vi "Write_para_port2_singalChange.vi"(8 "error in (no error)":errorcluster caption="错误输入（无错误）", 9 "索引":i32, 10 "布尔":bool=TRUE, 11 "address":i16=888 caption="地址" format="%.0x") -> (0 "error out":errorcluster caption="错误输出")   [LabVIEW 2011]
uses:
  <vilib>/Platform/portaccess.llb/In Port8.vi
  <vilib>/Platform/portaccess.llb/Out Port32.vi
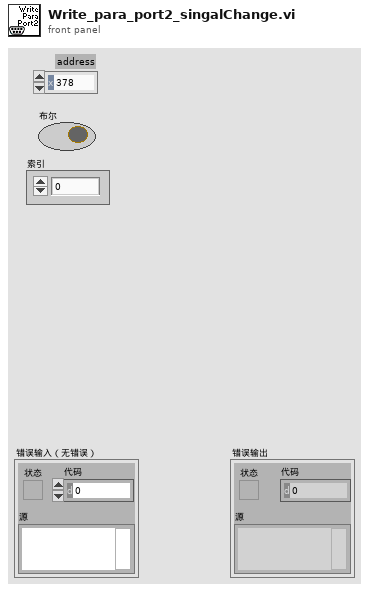
[diagram p1: front panel]
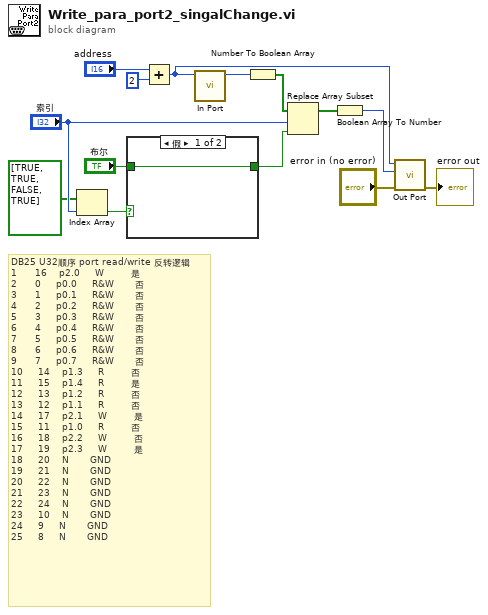
[diagram p0: block diagram]
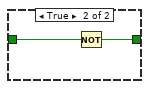
[diagram p2: hidden frame]
diagram:
  # "DB25\tU32顺序\tport\tread/write\t反转逻辑\n1\t     16\t   p2.0    \tW\t        是\n2\t     0    \tp0.0\t   \tR&W\t      否\n3\t     1\t\t   p0.1\t   \tR&W      \t否\n4\t\t    2\t   \tp0.2   \t\tR&W      \t否\n5\t\t    3\t\t   p0.3   \t\tR&W\t      否\n6\t\t    4\t   \tp0.4   \t\tR&W      \t否\n7\t\t    5\t   \tp0.5   \t\tR&W      \t否\n8\t\t    6\t   \tp0.6\t   \tR&W      \t否\n9\t    \t7\t   \tp0.7\t   \tR&W\t      否\n10\t    14   \tp1.3   \t\tR        \t否\n11\t   \t15   \tp1.4   \t\tR        \t是\n12\t   \t13   \tp1.2\t   \tR        \t否\n13    \t12   \tp1.1\t   \tR        \t否\n14     17   \tp2.1\t   \tW        \t是\n15    \t11   \tp1.0   \t\tR\t        否\n16    \t18   \tp2.2   \t\tW        \t否\n17    \t19\t   p2.3   \t\tW\t        是\n18    \t20   \tN   \t  \tGND\t\n19    \t21   \tN   \t  \tGND\t\n20\t    22\t   N\t  \t  \tGND\t\n21\t    23\t   N  \t  \t\tGND\t\n22\t    24\t   N  \t  \t\tGND\t\n23    \t10   \tN  \t  \t\tGND\t\n24    \t9\t    N  \t  \t\tGND\t\n25\t    8    \tN  \t  \t\tGND"
  n1 = Index Array(array=bool[] [TRUE, TRUE, FALSE, TRUE], index="索引") -> (element=w2:bool)
  n2 = case shown="假" w2 {
    tunnel: "布尔" -> [w15 w17]
    tunnel: [w15 w16] -> w1
    frame False {
    }
    frame True {
      n3 = Not(x=w17) -> (.not. x?=w16:bool)
    }
  }
  n4 = Add(x="address", y=i16 2) -> (x+y=w6:i16)
  n5 = call-poly <vilib>:"In Port.vi"("address"=w6) -> ("data read"=w12:i8)  [unwired: 7 in, 1 out]
  n6 = Number To Boolean Array(number=w12) -> (Boolean array=w11:bool[])
  n7 = Replace Array Subset(array=w11, new element=w1, index="索引") -> (w10:bool[])
  n8 = Boolean Array To Number(Boolean array=w10) -> (number=w9:u32)
  n9 = call-poly <vilib>:"Out Port.vi"("error in (no error)"="error in (no error)", "write value"=w9, "address"=w6) -> ("error out"=→"error out":errorcluster)  [unwired: 6 in]
